vi "Configure Filter (Line).vi"(7 "open?":bool, 8 "error in":errorcluster, 9 "frequency (kHz)":dbl=100.0 min=0.1 max=1000.0 step=0.1, 10 "channel":i32(ring) items=["All", "ELEM1", "ELEM2", "ELEM3", "ELEM4", "ELEM5", "ELEM6", "ELEM7"], 11 "VISA resource name":refnum<visa-resource-name>) -> (0 "error out":errorcluster, 3 "VISA resource out":refnum<visa-resource-name>)   [LabVIEW 2018, in "Suita SPAW7000.lvlib"]
uses:
  <instrlib>/Suita SPAW7000/Suita SPAW7000.lvlib
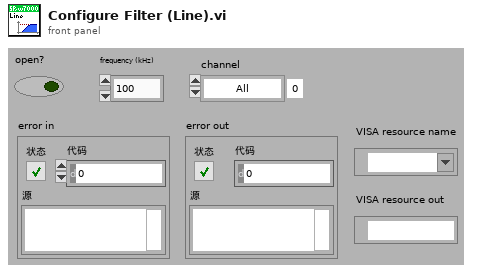
[diagram p1: front panel]
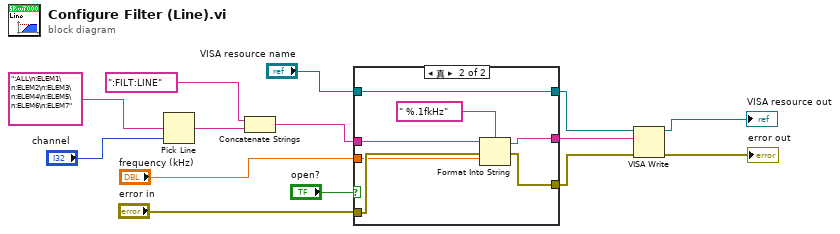
[diagram p0: block diagram]
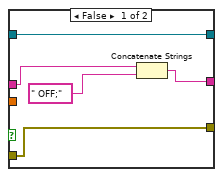
[diagram p2: hidden frame]
diagram:
  n1 = Pick Line ("ライン選択")(multi-line string=":ALL\n:ELEM1\n:ELEM2\n:ELEM3\n:ELEM4\n:ELEM5\n:ELEM6\n:ELEM7" ("複数行文字列"), line index="channel") -> (output string=w11:string)  [unwired: 1 out]
  n2 = Concatenate Strings(":FILT:LINE", w11) -> (w9:string)
  n3 = case shown="真" "open?" {
    tunnel: w9 -> [w18 w21]
    tunnel: [w16 w24] -> w7
    tunnel: [w17 w25] -> w6
    tunnel: "error in" -> [w16 w23]
    tunnel: "frequency (kHz)" -> [_ w22]
    tunnel: "VISA resource name" -> [w15 w20]
    tunnel: [w15 w20] -> w4
    frame False {
      n4 = Concatenate Strings(w18, " OFF;" ("文字列")) -> (w17:string)
    }
    frame True {
      n5 = Format Into String ("文字列にフォーマット")(format string=" %.1fkHz" ("形式文字列"), initial string=w21, error in=w23, w22) -> (resulting string=w25:string, error out=w24:errorcluster)
    }
  }
  n6 = VISA Write(VISA resource name=w4, write buffer=w6, error in (no error)=w7) -> (VISA resource name out=→"VISA resource out":refnum<visa-resource-name>, error out=→"error out":errorcluster)  [unwired: 1 out]
